vi "Load Instrument.Cryostat Classes.vi"(8 "error in (no error)":errorcluster, 11 "Control Experiment.lvclass":refnum<class "Control Experiment.lvclass">) -> (0 "error out":errorcluster, 3 "Control Experiment out":refnum<class "Control Experiment.lvclass">)   [LabVIEW 2016, in "Control Experiment.lvclass"]
uses:
  Control Experiment.lvclass
  <userlib>/LevyLab/Levylab Instruments/Instrument Types/Cryostat/Instrument.Cryostat.lvclass
  Control Experiment.lvclass/Control Experiment.ctl
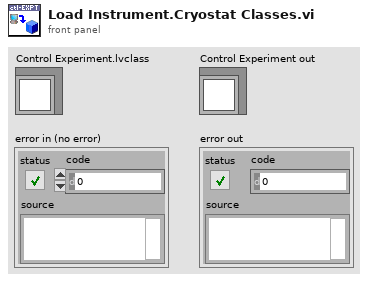
[diagram p1: front panel]
types:
  T1 = typedef "Control Experiment.lvclass/Instrument--enum.ctl" = enum16{"PPMS", "PPMS2", "MFP3D", "CYPHER", "THz1", "THz2", "MNK", "CF900", "JEOL", "AGILENT"}
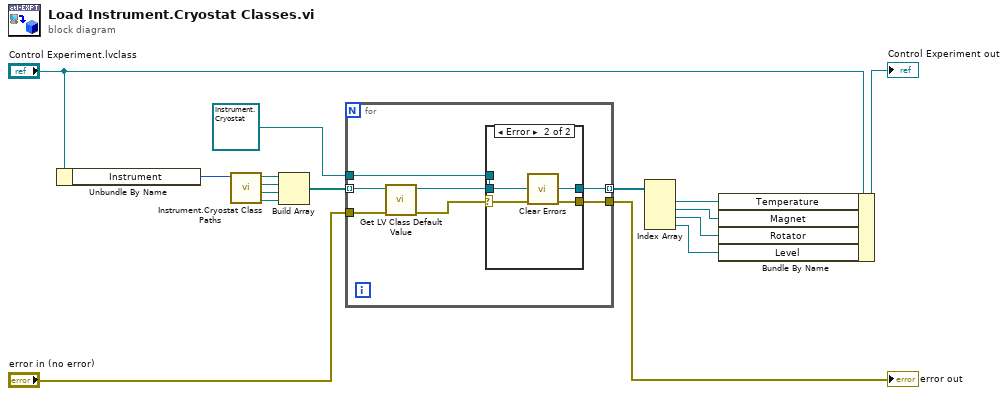
[diagram p0: block diagram]
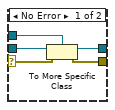
[diagram p2: hidden frame]
diagram:
  n1 = Unbundle By Name("Control Experiment.lvclass") -> ("Instrument"=w8:T1)
  n2 = call "Instrument.Cryostat Class Paths.vi"("instrument"=w8) -> ("Level Path"=w15:path, "Rotator Path"=w9:path, "Magnet Path"=w14:path, "Temperature Path"=w16:path)  [unwired: 3 in]
  n3 = Build Array(w16, w14, w9, w15) -> (w12:path[])
  n4 = for {
    tunnel: "error in (no error)" -> [w20]
    tunnel: refnum<class "Instrument.Cryostat.lvclass"> refnum ("Instruments.Level") -> [w19]
    tunnel: [w21] -> w7 mode=indexing
    tunnel: w12 -> [w18] mode=indexing
    tunnel: [w17] -> w11
    n5 = call <vilib>:"Get LV Class Default Value.vi"("error in (no error)"=w20, "class path"=w18) -> ("error out"=w22:errorcluster, "object"=w23:refnum<class>)  [unwired: 8 in]
    n6 = case shown="Error" w22 {
      selector: w22 -> [w25 w30]
      tunnel: [w28 w31] -> w21
      tunnel: w23 -> [w27 _]
      tunnel: [w26 w29] -> w17
      tunnel: w19 -> [w24 w31]
      frame No Error {
        n7 = To More Specific Class(target class=w24, reference=w27, error in=w25) -> (specific class reference=w28:refnum<class "Instrument.Cryostat.lvclass">, error out=w26:errorcluster)
      }
      frame Error {
        n8 = call <vilib>:"Clear Errors.vi"("error in (no error)"=w30) -> ("error out"=w29:errorcluster)  [unwired: 5 in, 1 out]
      }
    }
  }
  "error out" <- w11
  n9 = Index Array(array=w7) -> (element #1=w6:refnum<class "Instrument.Cryostat.lvclass">, element #2=w5:refnum<class "Instrument.Cryostat.lvclass">, element #3=w4:refnum<class "Instrument.Cryostat.lvclass">, element #4=w3:refnum<class "Instrument.Cryostat.lvclass">)  [unwired: 4 in]
  n10 = Bundle By Name(cluster="Control Experiment.lvclass", "Temperature"=w6, "Magnet"=w5, "Rotator"=w4, "Level"=w3) -> (→"Control Experiment out":refnum<class "Control Experiment.lvclass">)
